vi "global_rt_stream_connections.vi"() -> ()   [LabVIEW 2015]
uses:
  support_vis/message_queue/message_cluster.ctl
  support_vis/message_queue/message_queue.lvlib
panel:
  out "Connected？":bool caption="已连接？"
  in  "RT Stream Writer":refnum<k21> caption="RT网络流写入方端点"
  in  "RT Stream Reader":refnum<k21> caption="RT网络流读取方端点"
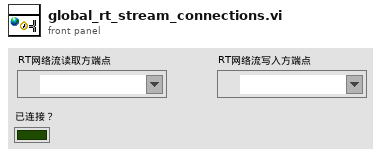
[diagram p1: front panel]
diagram:
